vi "Get Port Interface Name.vi"(8 "error in":errorcluster, 11 "Port Ref":T1 format="%.0x") -> (0 "error out":errorcluster, 1 "XNET Interface":refnum<k21>, 2 "CAN Interface Number":u16, 3 "Port Ref out":T1 format="%.0x")   [LabVIEW 2020, in "Communication Bus Template Scripting.lvlib"]
uses:
  Communication Bus Template Scripting.lvlib
  <vilib>/NI VeriStand/Custom Device API/Custom Device Item Ref.ctl
  Constants.vi
  <vilib>/NI VeriStand/Custom Device API/Get Item Property (U16).vi
  <vilib>/NI VeriStand/Custom Device API/Custom Device API.lvlib
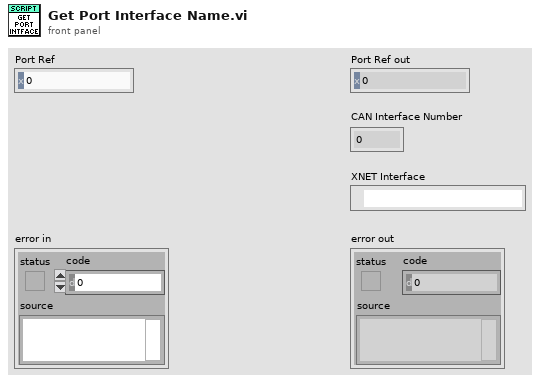
[diagram p1: front panel]
types:
  T1 = typedef "Custom Device API.lvlib/Custom Device Item Ref.ctl" = u64
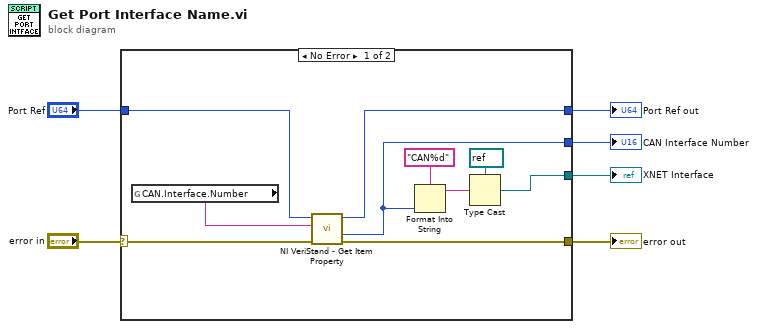
[diagram p0: block diagram]
diagram:
  n1 = case shown="No Error" "error in" {
    selector: "error in" -> [w14 w18]
    tunnel: "Port Ref" -> [w8 w17]
    tunnel: [w15 w18] -> w5
    tunnel: [w7 w17] -> w4
    tunnel: [w13 _] -> w2
    tunnel: [w9 _] -> w1
    frame No Error {
      n2 = global read "Constants.vi" "CAN.Interface.Number"() -> (w16:string)
      n3 = call-poly <vilib>:"NI VeriStand - Get Item Property.vi"("error in (no error)"=w14, "Property Name"=w16, "Item Ref in"=w8) -> ("error out"=w15:errorcluster, "Value"=w13:u16, "Item Ref out"=w7:T1)  [unwired: 5 in, 1 out]
      n4 = Format Into String(format string="CAN%d", w13) -> (resulting string=w11:string)  [unwired: 2 in, 1 out]
      n5 = Type Cast(type=refnum<k21> refnum ("XNET Interface"), x=w11) -> (*(type *) &x=w9:refnum<k21>)
    }
    frame Error {
    }
  }
  "error out" <- w5
  "CAN Interface Number" <- w2
  "Port Ref out" <- w4
  "XNET Interface" <- w1
